vi "Is Property Enum.vi"(8 "error in":errorcluster, 9 "Node":refnum<k20>) -> (0 "error out":errorcluster, 1 "Is Enum Property":bool, 2 "Enum Node":refnum<k20>)   [LabVIEW 2025]
uses:
  <resource>/objmgr/DOMUserDefRef.rc
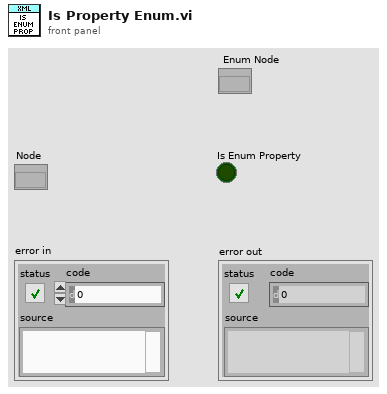
[diagram p1: front panel]
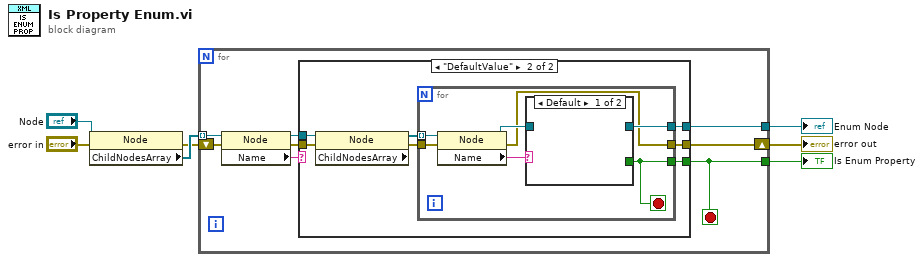
[diagram p0: block diagram]
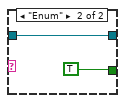
[diagram p3: hidden frame]
diagram:
  n1 = property class="Node"(reference="Node", error in="error in") -> (error out=w3:errorcluster, "ChildNodesArray"=w6:refnum<k20>[])  [unwired: 1 out]
  n2 = for {
    tunnel: w6 -> [w15] mode=indexing
    tunnel: [w12] -> w5
    tunnel: [w11] -> w4
    shift-right: [w8] -> w1
    shift-left: w3 -> [w10]
    stop <- w12 stop-if-true
    n3 = property class="Node"(reference=w15, error in=w10) -> (reference out=w13:refnum<k20>, error out=w9:errorcluster, "Name"=w14:string)
    n4 = case shown="\"DefaultValue\"" w14 {
      tunnel: w13 -> [_ w23]
      tunnel: [_ w21] -> w12
      tunnel: [_ w20] -> w11
      tunnel: w9 -> [w16 w19]
      tunnel: [w16 w17] -> w8
      frame Default {
      }
      frame "DefaultValue" {
        n5 = property class="Node"(reference=w23, error in=w19) -> (error out=w18:errorcluster, "ChildNodesArray"=w22:refnum<k20>[])  [unwired: 1 out]
        n6 = for {
          tunnel: w22 -> [w30] mode=indexing
          tunnel: [w24] -> w21
          tunnel: [w28] -> w20
          tunnel: w18 -> [w26]
          tunnel: [w25] -> w17
          stop <- w24 stop-if-true
          n7 = property class="Node"(reference=w30, error in=w26) -> (reference out=w27:refnum<k20>, error out=w25:errorcluster, "Name"=w29:string)
          n8 = case shown="Default" w29 {
            tunnel: [_ TRUE] -> w24
            tunnel: [_ w31] -> w28
            tunnel: w27 -> [_ w31]
            frame Default {
            }
            frame "Enum" {
            }
          }
        }
      }
    }
  }
  "error out" <- w1
  "Is Enum Property" <- w5
  "Enum Node" <- w4
